vi "increment date.vi"(8 "error in":errorcluster, 10 "# of Days":i32=1, 11 "Time Stamp In":timestamp=timestamp(3436645799.4727006 s since 1904-01-01)) -> (0 "error out":errorcluster, 3 "New Time Stamp":timestamp)   [LabVIEW 2013]
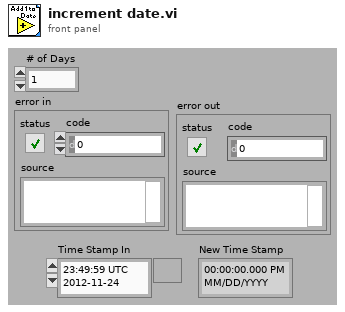
[diagram p1: front panel]
types:
  T1 = typedef "LVDateTimeRec.ctl" = cluster{"fractional second":dbl, "second":i32, "minute":i32, "hour":i32, "day of month":i32, "month":i32, "year":i32, "day of week":i32, "day of year":i32, "DST":i32}
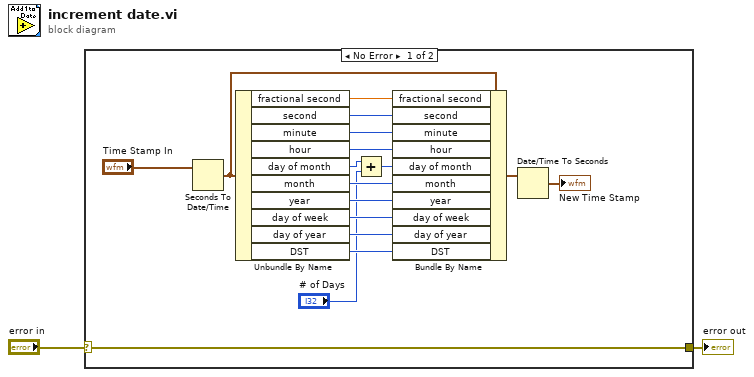
[diagram p0: block diagram]
diagram:
  n1 = case shown="No Error" "error in" {
    selector: "error in" -> [w3 w20]
    tunnel: [w3 w20] -> w1
    frame No Error {
      n2 = Seconds To Date/Time(time stamp (now)="Time Stamp In") -> (date time rec=w10:T1)  [unwired: 1 in]
      n3 = Unbundle By Name(w10) -> ("fractional second"=w19:dbl, "second"=w18:i32, "minute"=w17:i32, "hour"=w16:i32, "day of month"=w7:i32, "month"=w15:i32, "year"=w14:i32, "day of week"=w13:i32, "day of year"=w12:i32, "DST"=w11:i32)
      n4 = Add(x=w7, y="# of Days") -> (x+y=w6:i32)
      n5 = Bundle By Name(cluster=w10, "fractional second"=w19, "second"=w18, "minute"=w17, "hour"=w16, "day of month"=w6, "month"=w15, "year"=w14, "day of week"=w13, "day of year"=w12, "DST"=w11) -> (w9:T1)
      n6 = Date/Time To Seconds(2:w9) -> (0:→"New Time Stamp":timestamp)  [unwired: 1 in]
    }
    frame Error {
    }
  }
  "error out" <- w1
